vi "get_sensor_parameters_cluster.vi"(8 "error in (no error)":errorcluster, 10 "Sensor number":u8, 11 "VISA resource name":refnum<visa-resource-name>) -> (0 "error out":errorcluster, 2 "Sensor parameters":T1, 3 "VISA resource name out":refnum<visa-resource-name>)   [LabVIEW 2018]
doc: "Set the density of a material."
uses:
  Low Level/sensor_parameter_ring.ctl
  Low Level/sensor_parameters_strings.ctl
  Low Level/sensor_parameters.ctl
panel:
  in  "Sensor parameters (strings)":T2
  in  "Sensor parameter":T3 items=["Sensor Shutter Output", "Sensor Type", "Sensor Switch Output", "Auto-Z", "# of Positions", "# of Pulses", "Pulse On Time (s)", "Pulse Off Time (s)", "Recorder Output", "Recorder Function", "Recorder Range"]
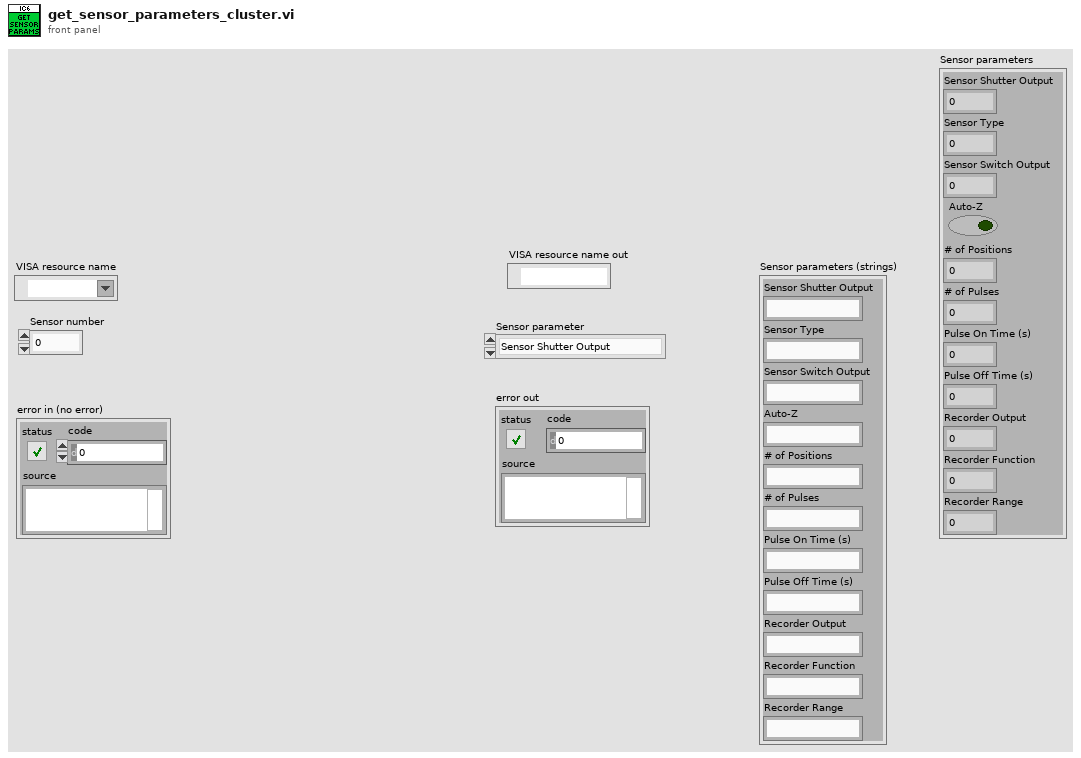
[diagram p1: front panel]
types:
  T1 = typedef "sensor_parameters.ctl" = cluster{"Sensor Shutter Output":u8, "Sensor Type":u8, "Sensor Switch Output":u8, "Auto-Z":bool, "# of Positions":u8, "# of Pulses":u8, "Pulse On Time (s)":sgl, "Pulse Off Time (s)":sgl, "Recorder Output":u8, "Recorder Function":u8, "Recorder Range":u32}
  T2 = typedef "sensor_parameters_strings.ctl" = cluster{"Sensor Shutter Output":string, "Sensor Type":string, "Sensor Switch Output":string, "Auto-Z":string, "# of Positions":string, "# of Pulses":string, "Pulse On Time (s)":string, "Pulse Off Time (s)":string, "Recorder Output":string, "Recorder Function":string, "Recorder Range":string}
  T3 = typedef "sensor_parameter_ring.ctl" = u16
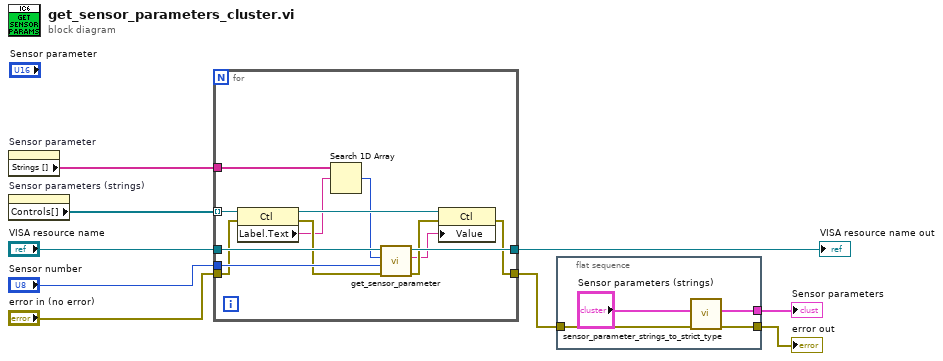
[diagram p0: block diagram]
diagram:
  n1 = property on="Sensor parameter" class="Ring (strict)"() -> ("Strings []"=w5:string[])  [unwired: 2 in, 2 out]
  n2 = property on="Sensor parameters (strings)" class="Clust (strict)"() -> ("Controls[]"=w1:refnum<vi>[])  [unwired: 2 in, 2 out]
  n3 = for {
    tunnel: "VISA resource name" -> [w22]
    tunnel: [w21] -> w8
    tunnel: [w13] -> w3
    tunnel: "error in (no error)" -> [w17]
    tunnel: "Sensor number" -> [w20]
    tunnel: w5 -> [w19]
    tunnel: w1 -> [w18] mode=indexing
    n4 = property class="Ctl"(reference=w18, error in=w17) -> (reference out=w15:refnum<vi>, error out=w16:errorcluster, "Label.Text"=w12:string)
    n5 = Search 1D Array(1D array=w19, element=w12) -> (index of element=w10:i32)  [unwired: 1 in]
    n6 = call "get_sensor_parameter.vi"("error in (no error)"=w16, "Sensor number"=w20, "Sensor parameter"=w10, "VISA resource name"=w22) -> ("error out"=w14:errorcluster, "Sensor parameter value"=w11:string, "VISA resource name out"=w21:refnum<visa-resource-name>)  [unwired: 5 in]
    n7 = property class="Ctl"(reference=w15, error in=w14, "Value"=w11) -> (error out=w13:errorcluster)  [unwired: 1 out]
  }
  "VISA resource name out" <- w8
  n8 = flat-sequence {
    tunnel: [w24] -> w4
    tunnel: w3 -> [w25]
    tunnel: [w23] -> w2
    frame #0 {
      n9 = call "sensor_parameter_strings_to_strict_type.vi"("error in (no error)"=w25, "Sensor parameters (strings)"="Sensor parameters (strings)") -> ("error out"=w24:errorcluster, "Sensor parameters"=w23:T1)  [unwired: 8 in]
    }
  }
  "error out" <- w4
  "Sensor parameters" <- w2
